vi "Open scan DB.vi"(4 "scan array":i32[](array[numeric]), 6 "End wavelength":dbl, 7 "Crop bottom":dbl, 8 "Start wavelength":dbl, 9 "delim":string=",", 10 "Crop top":i32, 11 "dup path":path) -> (0 "wavelengths":sgl[](array[numeric]), 3 "intensitites":sgl[][](array[numeric]))   [LabVIEW 2014]
uses:
  <vilib>/Utility/file.llb/Read From Spreadsheet File (DBL).vi
  Subs/Global 1.vi
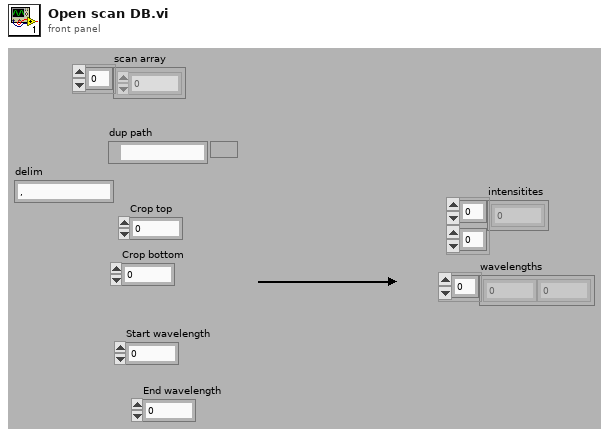
[diagram p1: front panel]
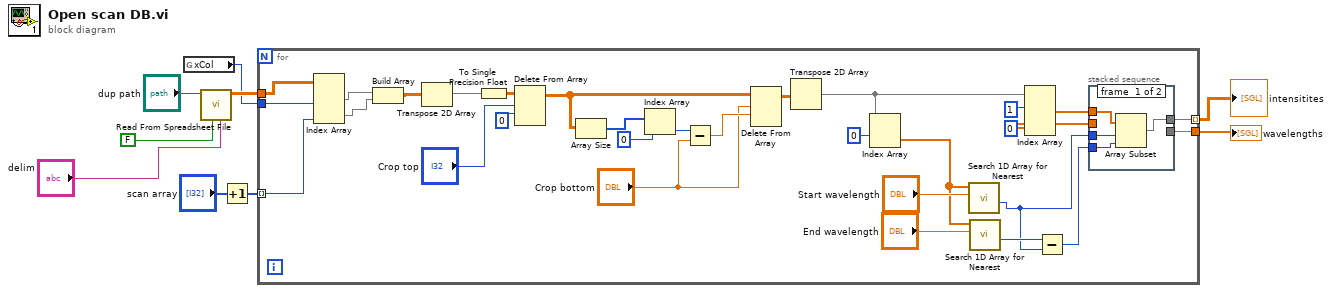
[diagram p0: block diagram]
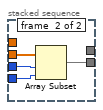
[diagram p2: hidden frame]
diagram:
  n1 = global read "Global 1.vi" "xCol"() -> (w1:i32)
  n2 = call-poly <vilib>:"Read From Spreadsheet File.vi"("delimiter (\\t)"="delim", "transpose (no:F)"=FALSE, "file path (dialog if empty)"="dup path") -> ("all rows"=w8:dbl[][])  [unwired: 4 in, 4 out]
  n3 = Increment(x="scan array") -> (x+1=w6:i32[])
  n4 = for {
    tunnel: [w37] -> w3 mode=indexing
    tunnel: [w36] -> w4
    tunnel: w8 -> [w21]
    tunnel: w6 -> [w17] mode=indexing
    tunnel: w1 -> [w10]
    n5 = Index Array(array=w21, index (col) #1=w10, index (col) #2=w17) -> (element #1=w16:dbl[], element #2=w18:dbl[])  [unwired: 2 in]
    n6 = Build Array(w16, w18) -> (w19:dbl[][])
    n7 = Transpose 2D Array(2D array=w19) -> (transposed array=w20:dbl[][])
    n8 = To Single Precision Float(number=w20) -> (single precision float=w39:sgl[][])
    n9 = Delete From Array(array=w39, length="Crop top", index (row)=0) -> (array with subset deleted=w24:sgl[][])  [unwired: 1 in, 1 out]
    n10 = Array Size(array=w24) -> (size(s)=w28:i32[])
    n11 = Index Array(array=w28, index=0) -> (element=w25:i32)
    n12 = Subtract(x=w25, y="Crop bottom") -> (x-y=w26:dbl)
    n13 = Delete From Array(array=w24, length="Crop bottom", index (row)=w26) -> (array with subset deleted=w29:sgl[][])  [unwired: 1 in, 1 out]
    n14 = Transpose 2D Array(2D array=w29) -> (transposed array=w40:sgl[][])
    n15 = Index Array(array=w40, index (row)=0) -> (element=w11:sgl[])  [unwired: 1 in]
    n16 = call "Search 1D Array for Nearest.vi"("desired element"="Start wavelength", "1D Array"=w11) -> ("closest index"=w12:i32)  [unwired: 8 in, 1 out]
    n17 = call "Search 1D Array for Nearest.vi"("desired element"="End wavelength", "1D Array"=w11) -> ("closest index"=w15:i32)  [unwired: 8 in, 1 out]
    n18 = Index Array(array=w40, index (row) #1=1 ("index (row)"), index (row) #2=0 ("index (row)")) -> (element #1=w34:sgl[], element #2=w35:sgl[])  [unwired: 2 in]
    n19 = Subtract(x=w15, y=w12) -> (x-y=w38:i32)
    n20 = stacked-sequence {
      tunnel: w34 -> [w44 _]
      tunnel: w12 -> [w43 w47]
      tunnel: w38 -> [w42 w46]
      tunnel: w35 -> [_ w48]
      tunnel: [_ w45] -> w36
      tunnel: [w41 _] -> w37
      frame #0 {
        n21 = Array Subset(array=w44, index=w43, length=w42) -> (w41:sgl[])
      }
      frame #1 {
        n22 = Array Subset(array=w48, index=w47, length=w46) -> (w45:sgl[])
      }
    }
  }
  "wavelengths" <- w4
  "intensitites" <- w3
